vi "Measure LTI ULS.vi"(8 "error in (no error)":errorcluster, 11 "LTI ULS Actor in":refnum<class "LTI ULS Actor.lvclass">) -> (0 "error out":errorcluster, 3 "LTI ULS Actor out":refnum<class "LTI ULS Actor.lvclass">)   [LabVIEW 2018, in "LTI ULS Actor.lvlib" / "LTI ULS Actor.lvclass"]
uses:
  LTI ULS Actor.lvclass
  C:/Users/dev/Documents/CODE/LabVIEW/microwaveverify/trunk/MWWL Verification/Sensor Actor/Sensor/Sensor.lvclass
  C:/Program Files (x86)/National Instruments/LabVIEW 2018/vi.lib/ActorFramework/Actor/Actor.lvclass
  Datalogger Actor/Data Record Control.ctl
  <vilib>/ActorFramework/Actor/Actor.lvclass/Actor.ctl
  MWWL Verification/MWWL Verification Messages/Send Value to Datalogger Msg/Send Value to Datalogger Msg.lvclass/Send Value to Datalogger Msg.ctl
  <vilib>/ActorFramework/Message Enqueuer/Message Enqueuer.lvclass/Message Enqueuer.ctl
  MWWL Verification/MWWL Verification Messages/Log Event Msg/Log Event Msg.lvclass/Log Event Msg.ctl
  <vilib>/ActorFramework/Message Enqueuer/Enqueue.vi
  MWWL Verification/MWWL Verification Messages/Send Value to Datalogger Msg/Send Value to Datalogger Msg.lvclass
  C:/Program Files (x86)/National Instruments/LabVIEW 2018/vi.lib/ActorFramework/Message/Message.lvclass
  MWWL Verification/MWWL Verification Messages/Log Event Msg/Log Event Msg.lvclass
  <vilib>/ActorFramework/Message Priority Queue/Priority Enqueue.vi
  <vilib>/ActorFramework/Actor/Actor.lvclass
  Sensor Actor/Sensor/Sensor.lvclass
  Datalogger Actor/Datalogger Actor.lvclass
panel:
  in  "Data Record":T1
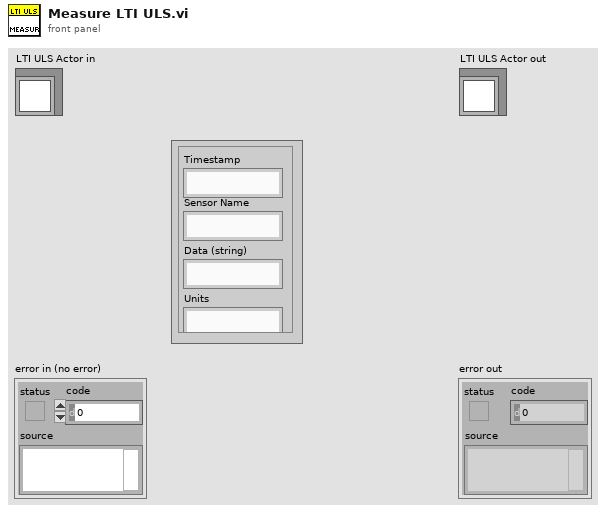
[diagram p1: front panel]
types:
  T1 = typedef "Datalogger.lvlib/Datalogger Actor.lvclass/Data Record Control.ctl" = cluster{"Timestamp":string, "Sensor Name":string, "Data (string)":string, "Units":string}
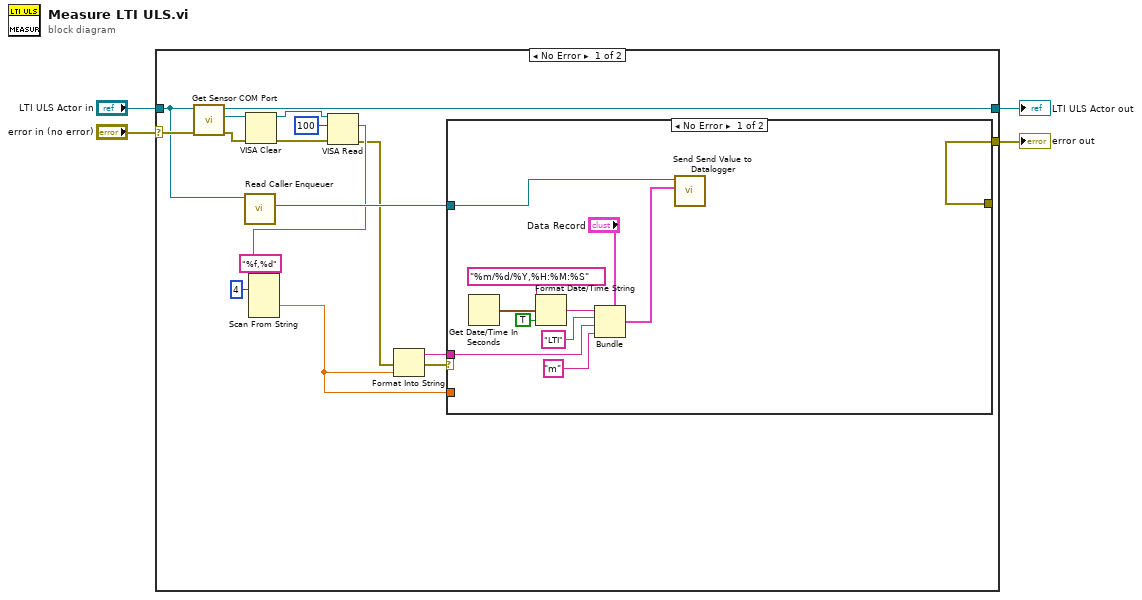
[diagram p0: block diagram]
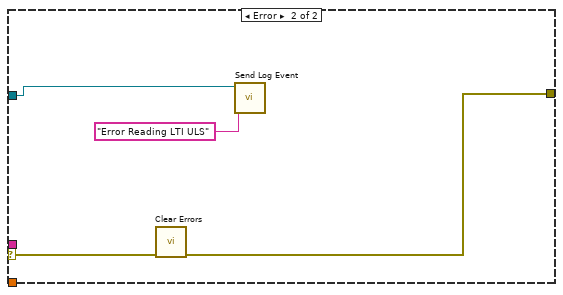
[diagram p2: hidden frame]
diagram:
  n1 = case shown="No Error" "error in (no error)" {
    selector: "error in (no error)" -> [w16 w37]
    tunnel: [w14 w37] -> w3
    tunnel: [w15 w36] -> w1
    tunnel: "LTI ULS Actor in" -> [w12 w36]
    frame No Error {
      n2 = call "Get Sensor COM Port.vi"("error in (no error)"=w16, "Sensor in"=w12) -> ("error out"=w19:errorcluster, "COM Port"=w20:refnum<visa-resource-name>, "Sensor out"=w15:refnum<class "LTI ULS Actor.lvclass">)  [unwired: 7 in]
      n3 = call <vilib>:"Read Caller Enqueuer.vi"("Actor"=w12) -> ("Caller Enqueuer"=w10:refnum<class "Message Enqueuer.lvclass">)  [unwired: 10 in]
      n4 = VISA Clear(VISA resource name=w20, error in (no error)=w19) -> (VISA resource name out=w18:refnum<visa-resource-name>, error out=w17:errorcluster)
      n5 = VISA Read(VISA resource name=w18, byte count=u32 100, error in (no error)=w17) -> (read buffer=w9:string, error out=w7:errorcluster)  [unwired: 2 out]
      n6 = Scan From String(format string="%f,%d", input string=w9, initial scan location=u32 4) -> (output 1=w5:dbl)  [unwired: 4 in, 3 out]
      n7 = Format Into String(error in=w7, w5) -> (resulting string=w8:string, error out=w6:errorcluster)  [unwired: 2 in]
      n8 = case shown="No Error" w6 {
        selector: w6 -> [_ w35]
        tunnel: [_ w34] -> w14
        tunnel: w10 -> [w23 w32]
        tunnel: w8 -> [w22 _]
        tunnel: w5 -> [_ _]
        frame No Error {
          n9 = Get Date/Time In Seconds() -> (seconds since 1Jan1904=w26:timestamp)
          n10 = Format Date/Time String(time format string (%c)="%m/%d/%Y,%H:%M:%S", seconds (now)=w26, UTC format=TRUE) -> (date/time string=w28:string)
          n11 = Bundle(cluster="Data Record", "Timestamp"=w28, "Sensor Name"="LTI" ("time format string (%c)"), "Data (string)"=w22, "Units"="m" ("time format string (%c)")) -> (w24:T1)
          n12 = call "Send Send Value to Datalogger.vi"("Data Record"=w24, "Message Enqueuer in"=w23) -> ()  [unwired: 8 in, 2 out]
        }
        frame Error {
          n13 = call <vilib>:"Clear Errors.vi"("error in (no error)"=w35) -> ("error out"=w34:errorcluster)  [unwired: 5 in, 1 out]
          n14 = call "Send Log Event.vi"("Event Text"="Error Reading LTI ULS", "Message Enqueuer"=w32) -> ()  [unwired: 8 in, 2 out]
        }
      }
    }
    frame Error {
    }
  }
  "error out" <- w3
  "LTI ULS Actor out" <- w1
